vi "Диапазоны Delta.vi"(0 "Вип":dbl[](array[numeric]), 1 "Пересчет":dbl[](array[numeric]), 2 "Atm":dbl[](array[numeric]), 3 "Время":dbl[](array[numeric]), 4 "Temper":dbl=25.0) -> (5 "output cluster":cluster{"Время":dbl[], dbl[]}, 6 "appended array":dbl[](array[numeric]), 8 "Диапазон":dbl=1.0, 9 "Q":dbl)   [LabVIEW 2018]
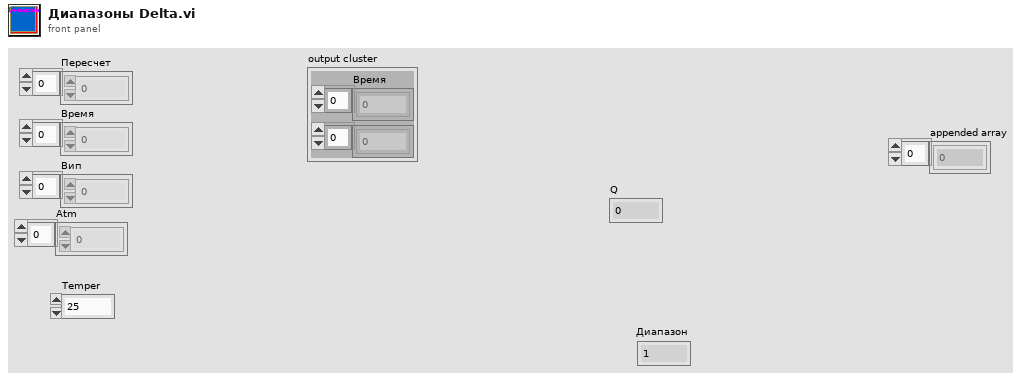
[diagram p1: front panel]
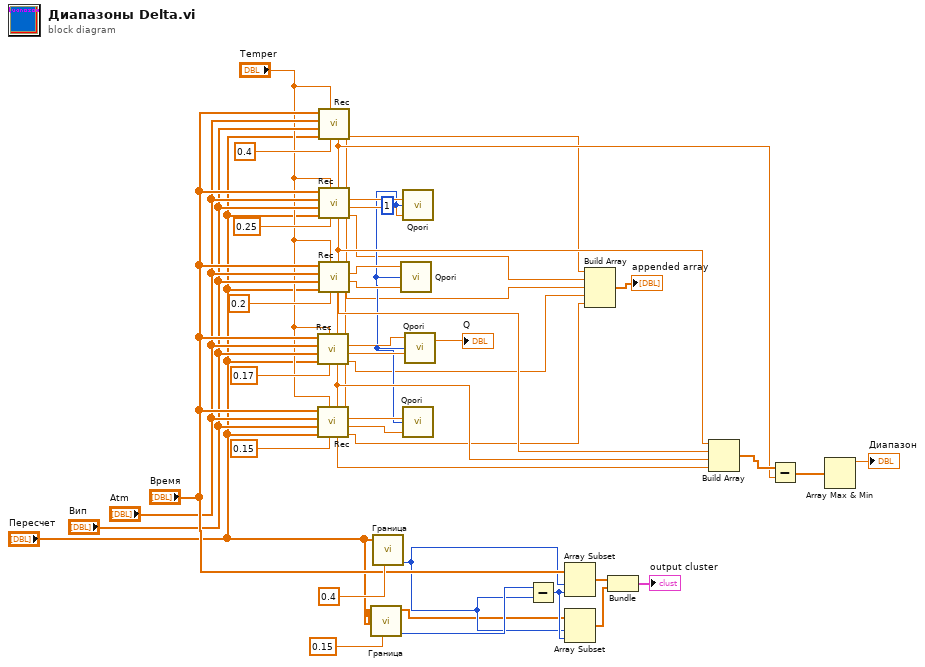
[diagram p0: block diagram]
diagram:
  w7 = 1 ("Numeric")
  n1 = call "Rec.vi"("Граница"=0.4, "Temper"="Temper", "Пересчет"="Пересчет", "Вип"="Вип", "Atm"="Atm", "Время"="Время") -> ("n"=w6:dbl, "time"=w31:dbl)  [unwired: 2 in, 2 out]
  n2 = call "Rec.vi"("N"=w6, "t"=w31, "Граница"=0.25, "Temper"="Temper", "Пересчет"="Пересчет", "Вип"="Вип", "Atm"="Atm", "Время"="Время") -> ("n"=w5:dbl, "DT"=w29:dbl, "раз"=w30:dbl, "time"=w10:dbl)
  n3 = call "Rec.vi"("N"=w5, "t"=w10, "Граница"=0.2, "Temper"="Temper", "Пересчет"="Пересчет", "Вип"="Вип", "Atm"="Atm", "Время"="Время") -> ("n"=w4:dbl, "DT"=w26:dbl, "раз"=w27:dbl, "time"=w11:dbl)
  n4 = call "Rec.vi"("N"=w4, "t"=w11, "Граница"=0.17, "Temper"="Temper", "Пересчет"="Пересчет", "Вип"="Вип", "Atm"="Atm", "Время"="Время") -> ("n"=w3:dbl, "DT"=w24:dbl, "раз"=w25:dbl, "time"=w12:dbl)
  n5 = call "Rec.vi"("N"=w3, "t"=w12, "Граница"=0.15, "Temper"="Temper", "Пересчет"="Пересчет", "Вип"="Вип", "Atm"="Atm", "Время"="Время") -> ("n"=w2:dbl, "DT"=w16:dbl, "раз"=w17:dbl, "time"=w13:dbl)
  n6 = call "Граница.vi"("Перерасчет"="Пересчет", "Граница"=0.15 ("element")) -> ("Numeric 4"=w33:i32)  [unwired: 3 in, 3 out]
  n7 = call "Граница.vi"("Перерасчет"="Пересчет", "Граница"=0.4 ("element")) -> ("Numeric 4"=w9:i32)  [unwired: 3 in, 3 out]
  n8 = call "Qpori.vi"("Dt"=w26, "Numeric"=w7, "Dn"=w27) -> ()  [unwired: 2 out]
  n9 = call "Qpori.vi"("Dt"=w29, "Numeric"=w7, "Dn"=w30) -> ()  [unwired: 2 out]
  n10 = call "Qpori.vi"("Dt"=w16, "Numeric"=w7, "Dn"=w17) -> ()  [unwired: 2 out]
  n11 = call "Qpori.vi"("Dt"=w24, "Numeric"=w7, "Dn"=w25) -> ("Q"=→"Q":dbl)  [unwired: 1 out]
  n12 = Subtract(x=w33, y=w9) -> (x-y=w35:i32)
  n13 = Array Subset(array="Время", index=w9, length=w35) -> (w36:dbl[])
  n14 = Array Subset(array="Пересчет", index=w9, length=w35) -> (w42:dbl[])
  n15 = Build Array(w6, w5, w4, w3, w2) -> (→"appended array":dbl[])
  n16 = Bundle(w36, w42) -> (→"output cluster":cluster{dbl[], dbl[]})  [unwired: 1 in]
  n17 = Build Array(w10, w11, w12, w13) -> (w38:dbl[])
  n18 = Subtract(x=w38, y=w31) -> (x-y=w37:dbl[])
  n19 = Array Max & Min(array=w37) -> (max value=→"Диапазон":dbl)  [unwired: 3 out]
